vi "DataClusterDestroy.vi"(8 "error in (no error)":errorcluster) -> (0 "error out":errorcluster)   [LabVIEW 2013, in "Data.lvclass"]
uses:
  Data.lvclass
  Singleton.lvclass/Destructor.vi
  Singleton.lvclass/Constructor.vi
  Singleton.lvclass/Singleton.lvclass
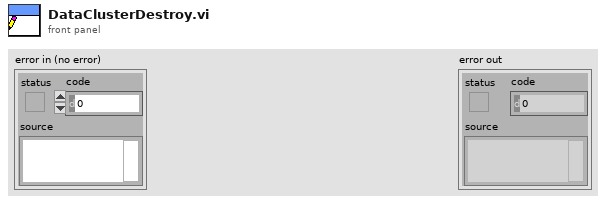
[diagram p1: front panel]
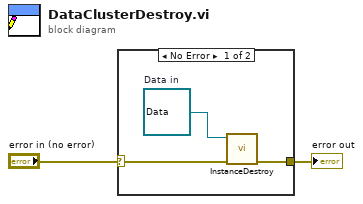
[diagram p0: block diagram]
diagram:
  n1 = case shown="No Error" "error in (no error)" {
    selector: "error in (no error)" -> [w4 w6]
    tunnel: [w3 w6] -> w1
    frame No Error {
      w5 = refnum<class "Data.lvclass"> refnum  # Data in
      n2 = call "InstanceDestroy.vi"("error in (no error)"=w4, "Singleton.lvclass In"=w5) -> ("error out"=w3:errorcluster)  [unwired: 8 in, 1 out]
    }
    frame Error {
    }
  }
  "error out" <- w1
